vi "Zernike_gen.vi"(8 "Coefficient":dbl[](array[numeric]), 9 "Gray level max":i32=255, 10 "dimension size y":i32=1024, 11 "dimension size x":i32=1280) -> (3 "mask":dbl[][](array[numeric]))   [LabVIEW 2020]
panel:
  out "theta":u8[][](array[numeric])
  out "rho":u8[][](array[numeric])
  out "X":u8[][](array[numeric])
  out "Y":u8[][](array[numeric])
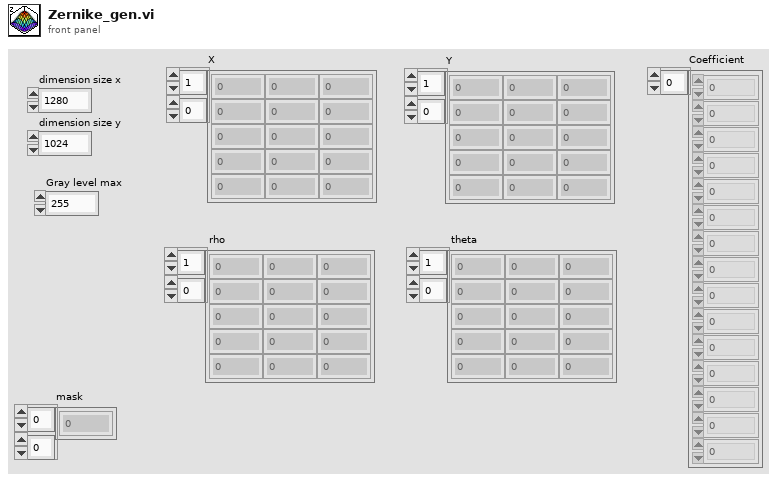
[diagram p1: front panel]
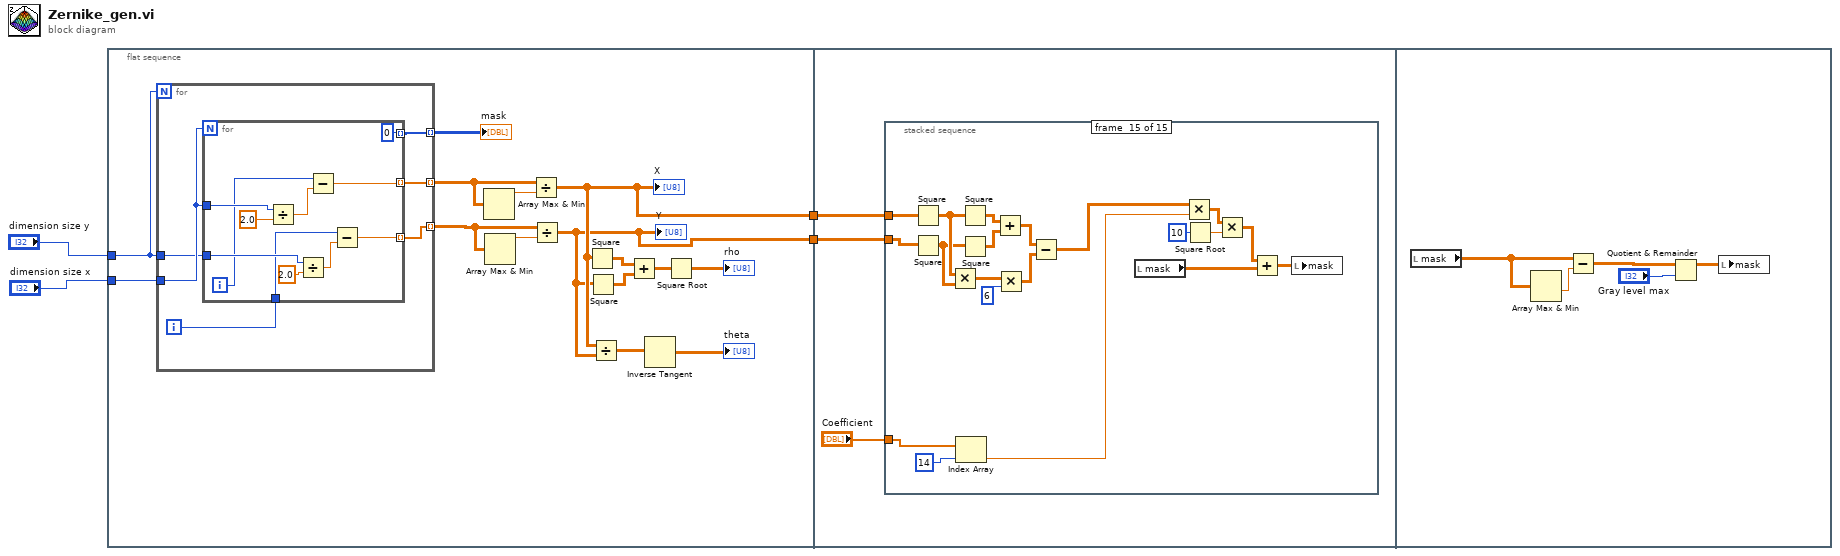
[diagram p0: block diagram]
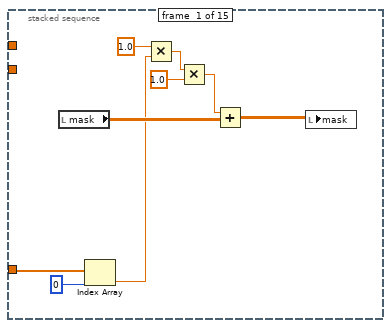
[diagram p2: hidden frame]
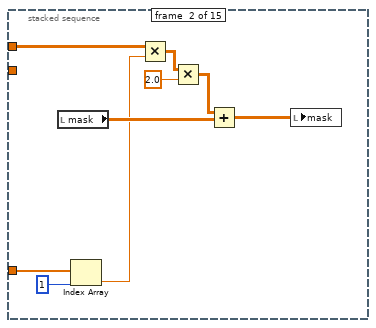
[diagram p3: hidden frame]
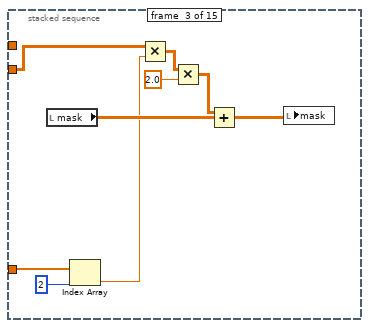
[diagram p4: hidden frame]
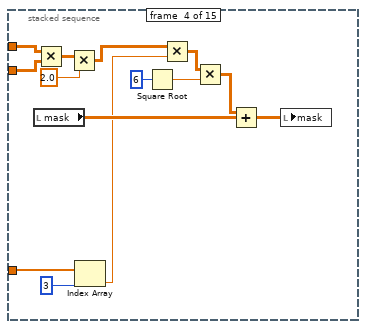
[diagram p5: hidden frame]
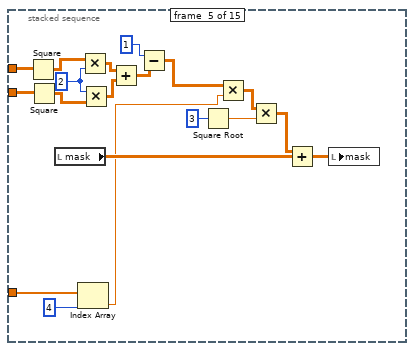
[diagram p6: hidden frame]
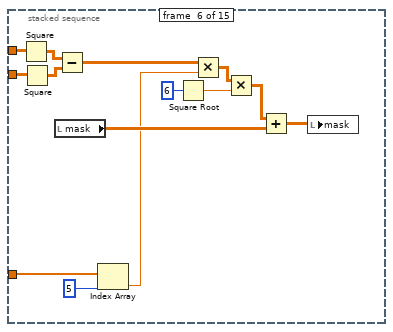
[diagram p7: hidden frame]
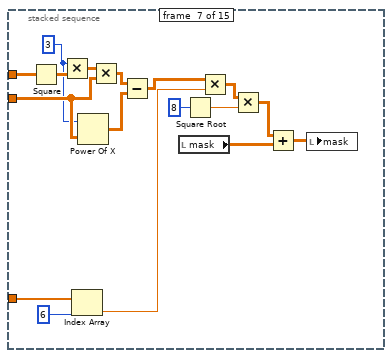
[diagram p8: hidden frame]
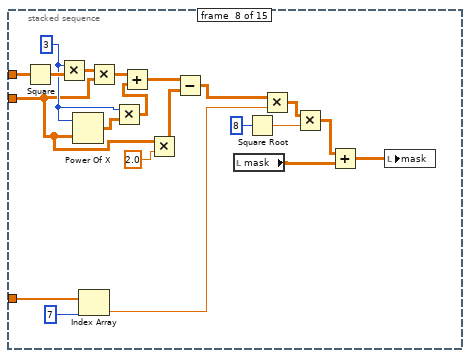
[diagram p9: hidden frame]
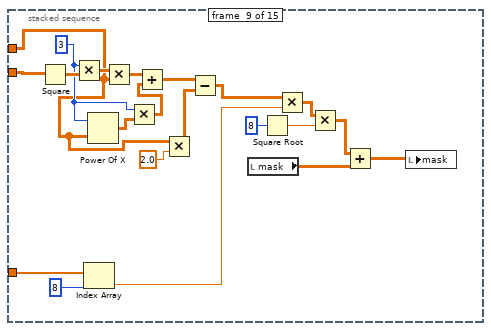
[diagram p10: hidden frame]
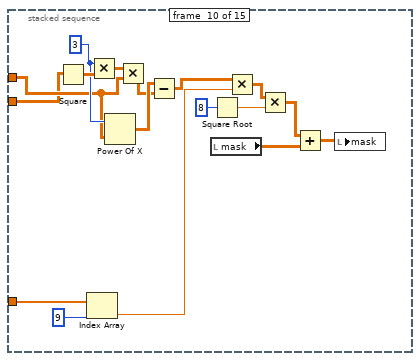
[diagram p11: hidden frame]
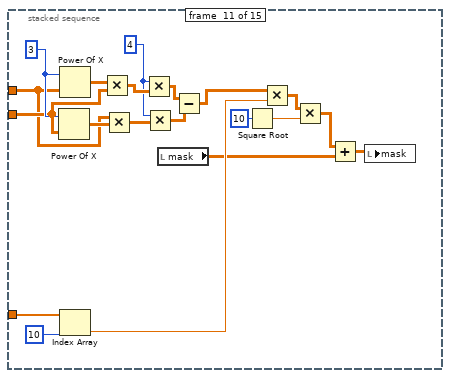
[diagram p12: hidden frame]
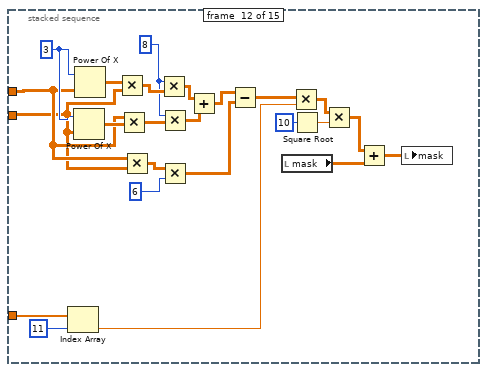
[diagram p13: hidden frame]
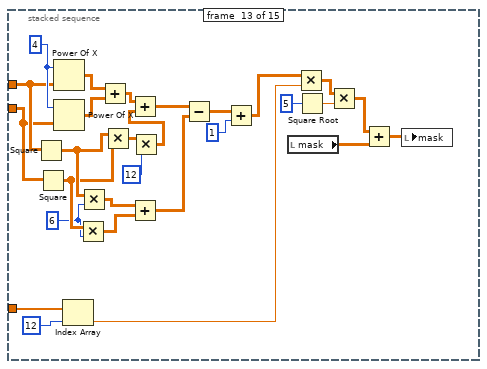
[diagram p14: hidden frame]
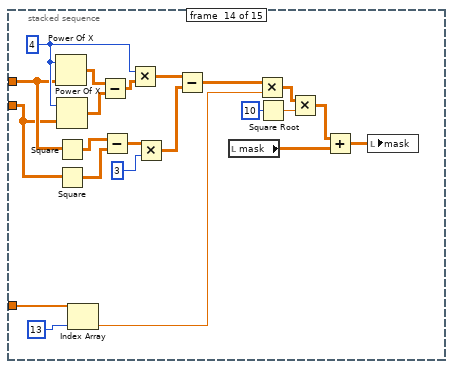
[diagram p15: hidden frame]
diagram:
  n1 = flat-sequence {
    tunnel: [w6] -> w4
    tunnel: [w5] -> w3
    tunnel: "dimension size x" -> [w19]
    tunnel: "dimension size y" -> [w15]
    tunnel: w4 -> [w39]
    tunnel: w3 -> [w37]
    frame #0 {
      n2 = for {
        N: w15 -> [_]
        tunnel: [w25] -> w10 mode=indexing
        tunnel: w19 -> [w22]
        tunnel: [w23] -> w12 mode=indexing
        tunnel: w15 -> [w21]
        tunnel: [w20] -> w9 mode=indexing
        i -> [w24]
        n3 = for {
          N: w22 -> [_]
          tunnel: [w28] -> w25 mode=indexing
          tunnel: w24 -> [w29]
          tunnel: [w33] -> w23 mode=indexing
          tunnel: w22 -> [w35]
          tunnel: w21 -> [w31]
          tunnel: [0] -> w20 mode=indexing
          i -> [w27]
          n4 = Divide(x=w35, y=2.0) -> (x/y=w34:dbl)
          n5 = Divide(x=w31, y=2.0) -> (x/y=w30:dbl)
          n6 = Subtract(x=w27, y=w34) -> (x-y=w33:dbl)
          n7 = Subtract(x=w29, y=w30) -> (x-y=w28:dbl)
        }
      }
      "mask" <- w9
      n8 = Array Max & Min(array=w12) -> (max value=w13:dbl)  [unwired: 3 out]
      n9 = Array Max & Min(array=w10) -> (max value=w11:dbl)  [unwired: 3 out]
      n10 = Divide(x=w12, y=w13) -> (x/y=w6:dbl[][])
      "X" <- w6
      n11 = Divide(x=w10, y=w11) -> (x/y=w5:dbl[][])
      "Y" <- w5
      n12 = Square(x=w6) -> (x^2=w18:dbl[][])
      n13 = Square(x=w5) -> (x^2=w17:dbl[][])
      n14 = Divide(x=w6, y=w5) -> (x/y=w14:dbl[][])
      n15 = Add(x=w18, y=w17) -> (x+y=w16:dbl[][])
      n16 = Inverse Tangent(1:w14) -> (0:→"theta":dbl[][])
      n17 = Square Root(x=w16) -> (sqrt(x)=→"rho":dbl[][])
    }
    frame #1 {
      n18 = stacked-sequence {
        tunnel: w39 -> [_ w53 _ w78 w95 w109 w126 w147 w157 w181 w200 w221 w254 w275 w298]
        tunnel: "Coefficient" -> [w47 w54 w59 w68 w82 w101 w117 w132 w155 w176 w194 w213 w237 w265 w287]
        tunnel: w37 -> [_ _ w61 w77 w94 w108 w122 w139 w158 w180 w203 w220 w253 w274 w297]
        frame #0 {
          n19 = local read "mask"() -> (w43:dbl[][])
          n20 = Index Array(array=w47, index=0) -> (element=w40:dbl)
          n21 = Multiply(x=1.0, y=w40) -> (x*y=w45:dbl)
          n22 = Multiply(x=w45, y=1.0) -> (x*y=w46:dbl)
          n23 = Add(x=w46, y=w43) -> (x+y=w42:dbl[][])
          n24 = local write "mask"(w42) -> ()
        }
        frame #1 {
          n25 = local read "mask"() -> (w55:dbl[][])
          n26 = Index Array(array=w54, index=1) -> (element=w52:dbl)
          n27 = Multiply(x=w53, y=w52) -> (x*y=w50:dbl[][])
          n28 = Multiply(x=w50, y=2.0) -> (x*y=w49:dbl[][])
          n29 = Add(x=w49, y=w55) -> (x+y=w56:dbl[][])
          n30 = local write "mask"(w56) -> ()
        }
        frame #2 {
          n31 = local read "mask"() -> (w63:dbl[][])
          n32 = Index Array(array=w59, index=2) -> (element=w58:dbl)
          n33 = Multiply(x=w61, y=w58) -> (x*y=w65:dbl[][])
          n34 = Multiply(x=w65, y=2.0) -> (x*y=w66:dbl[][])
          n35 = Add(x=w66, y=w63) -> (x+y=w62:dbl[][])
          n36 = local write "mask"(w62) -> ()
        }
        frame #3 {
          n37 = local read "mask"() -> (w71:dbl[][])
          n38 = Multiply(x=w78, y=w77) -> (x*y=w75:dbl[][])
          n39 = Multiply(x=w75, y=2.0) -> (x*y=w74:dbl[][])
          n40 = Index Array(array=w68, index=3) -> (element=w67:dbl)
          n41 = Square Root(x=6) -> (sqrt(x)=w72:dbl)
          n42 = Multiply(x=w74, y=w67) -> (x*y=w80:dbl[][])
          n43 = Multiply(x=w80, y=w72) -> (x*y=w79:dbl[][])
          n44 = Add(x=w79, y=w71) -> (x+y=w70:dbl[][])
          n45 = local write "mask"(w70) -> ()
        }
        frame #4 {
          w91 = 2
          n46 = Square(x=w95) -> (x^2=w93:dbl[][])
          n47 = Square(x=w94) -> (x^2=w92:dbl[][])
          n48 = local read "mask"() -> (w85:dbl[][])
          n49 = Index Array(array=w82, index=4) -> (element=w81:dbl)
          n50 = Multiply(x=w93, y=w91) -> (x*y=w90:dbl[][])
          n51 = Multiply(x=w91, y=w92) -> (x*y=w89:dbl[][])
          n52 = Add(x=w90, y=w89) -> (x+y=w88:dbl[][])
          n53 = Subtract(x=1, y=w88) -> (x-y=w86:dbl[][])
          n54 = Square Root(x=3) -> (sqrt(x)=w99:dbl)
          n55 = Multiply(x=w86, y=w81) -> (x*y=w97:dbl[][])
          n56 = Multiply(x=w97, y=w99) -> (x*y=w98:dbl[][])
          n57 = Add(x=w98, y=w85) -> (x+y=w84:dbl[][])
          n58 = local write "mask"(w84) -> ()
        }
        frame #5 {
          n59 = Square(x=w109) -> (x^2=w107:dbl[][])
          n60 = Square(x=w108) -> (x^2=w106:dbl[][])
          n61 = local read "mask"() -> (w104:dbl[][])
          n62 = Subtract(x=w107, y=w106) -> (x-y=w105:dbl[][])
          n63 = Index Array(array=w101, index=5) -> (element=w100:dbl)
          n64 = Square Root(x=6) -> (sqrt(x)=w111:dbl)
          n65 = Multiply(x=w105, y=w100) -> (x*y=w113:dbl[][])
          n66 = Multiply(x=w113, y=w111) -> (x*y=w112:dbl[][])
          n67 = Add(x=w112, y=w104) -> (x+y=w103:dbl[][])
          n68 = local write "mask"(w103) -> ()
        }
        frame #6 {
          w121 = 3
          n69 = Square(x=w126) -> (x^2=w125:dbl[][])
          n70 = Multiply(x=w121, y=w125) -> (x*y=w124:dbl[][])
          n71 = Index Array(array=w117, index=6) -> (element=w116:dbl)
          n72 = Power Of X(1:w122, 2:w121) -> (0:w120:dbl[][])
          n73 = Multiply(x=w124, y=w122) -> (x*y=w123:dbl[][])
          n74 = Subtract(x=w123, y=w120) -> (x-y=w119:dbl[][])
          n75 = local read "mask"() -> (w115:dbl[][])
          n76 = Square Root(x=8) -> (sqrt(x)=w130:dbl)
          n77 = Multiply(x=w119, y=w116) -> (x*y=w128:dbl[][])
          n78 = Multiply(x=w128, y=w130) -> (x*y=w129:dbl[][])
          n79 = Add(x=w129, y=w115) -> (x+y=w114:dbl[][])
          n80 = local write "mask"(w114) -> ()
        }
        frame #7 {
          w142 = 3
          n81 = Square(x=w147) -> (x^2=w146:dbl[][])
          n82 = Multiply(x=w142, y=w146) -> (x*y=w145:dbl[][])
          n83 = Power Of X(1:w139, 2:w142) -> (0:w143:dbl[][])
          n84 = Index Array(array=w132, index=7) -> (element=w131:dbl)
          n85 = Multiply(x=w145, y=w139) -> (x*y=w144:dbl[][])
          n86 = Multiply(x=w142, y=w143) -> (x*y=w141:dbl[][])
          n87 = Add(x=w144, y=w141) -> (x+y=w137:dbl[][])
          n88 = Multiply(x=w139, y=2.0) -> (x*y=w138:dbl[][])
          n89 = Subtract(x=w137, y=w138) -> (x-y=w136:dbl[][])
          n90 = local read "mask"() -> (w135:dbl[][])
          n91 = Square Root(x=8) -> (sqrt(x)=w151:dbl)
          n92 = Multiply(x=w136, y=w131) -> (x*y=w149:dbl[][])
          n93 = Multiply(x=w149, y=w151) -> (x*y=w150:dbl[][])
          n94 = Add(x=w150, y=w135) -> (x+y=w134:dbl[][])
          n95 = local write "mask"(w134) -> ()
        }
        frame #8 {
          w160 = 3
          n96 = Square(x=w158) -> (x^2=w165:dbl[][])
          n97 = Multiply(x=w160, y=w165) -> (x*y=w166:dbl[][])
          n98 = Index Array(array=w155, index=8) -> (element=w154:dbl)
          n99 = Power Of X(1:w157, 2:w160) -> (0:w168:dbl[][])
          n100 = Multiply(x=w166, y=w157) -> (x*y=w167:dbl[][])
          n101 = Multiply(x=w160, y=w168) -> (x*y=w169:dbl[][])
          n102 = Add(x=w167, y=w169) -> (x+y=w171:dbl[][])
          n103 = Multiply(x=w157, y=2.0) -> (x*y=w170:dbl[][])
          n104 = Subtract(x=w171, y=w170) -> (x-y=w172:dbl[][])
          n105 = local read "mask"() -> (w153:dbl[][])
          n106 = Square Root(x=8) -> (sqrt(x)=w162:dbl)
          n107 = Multiply(x=w172, y=w154) -> (x*y=w164:dbl[][])
          n108 = Multiply(x=w164, y=w162) -> (x*y=w163:dbl[][])
          n109 = Add(x=w163, y=w153) -> (x+y=w152:dbl[][])
          n110 = local write "mask"(w152) -> ()
        }
        frame #9 {
          w182 = 3
          n111 = Square(x=w180) -> (x^2=w187:dbl[][])
          n112 = Index Array(array=w176, index=9) -> (element=w175:dbl)
          n113 = Multiply(x=w182, y=w187) -> (x*y=w188:dbl[][])
          n114 = Power Of X(1:w181, 2:w182) -> (0:w179:dbl[][])
          n115 = Multiply(x=w188, y=w181) -> (x*y=w178:dbl[][])
          n116 = Subtract(x=w179, y=w178) -> (x-y=w189:dbl[][])
          n117 = local read "mask"() -> (w174:dbl[][])
          n118 = Square Root(x=8) -> (sqrt(x)=w184:dbl)
          n119 = Multiply(x=w189, y=w175) -> (x*y=w186:dbl[][])
          n120 = Multiply(x=w186, y=w184) -> (x*y=w185:dbl[][])
          n121 = Add(x=w185, y=w174) -> (x+y=w173:dbl[][])
          n122 = local write "mask"(w173) -> ()
        }
        frame #10 {
          w198 = 4
          w205 = 3
          n123 = Power Of X(1:w203, 2:w205) -> (0:w201:dbl[][])
          n124 = Power Of X(1:w200, 2:w205) -> (0:w204:dbl[][])
          n125 = Index Array(array=w194, index=10) -> (element=w193:dbl)
          n126 = Multiply(x=w204, y=w203) -> (x*y=w202:dbl[][])
          n127 = Multiply(x=w200, y=w201) -> (x*y=w199:dbl[][])
          n128 = Multiply(x=w198, y=w202) -> (x*y=w197:dbl[][])
          n129 = Multiply(x=w198, y=w199) -> (x*y=w192:dbl[][])
          n130 = local read "mask"() -> (w191:dbl[][])
          n131 = Subtract(x=w197, y=w192) -> (x-y=w196:dbl[][])
          n132 = Square Root(x=10) -> (sqrt(x)=w209:dbl)
          n133 = Multiply(x=w196, y=w193) -> (x*y=w207:dbl[][])
          n134 = Multiply(x=w207, y=w209) -> (x*y=w208:dbl[][])
          n135 = Add(x=w208, y=w191) -> (x+y=w190:dbl[][])
          n136 = local write "mask"(w190) -> ()
        }
        frame #11 {
          w222 = 8
          w223 = 3
          n137 = Index Array(array=w213, index=11) -> (element=w212:dbl)
          n138 = Power Of X(1:w220, 2:w223) -> (0:w226:dbl[][])
          n139 = Power Of X(1:w221, 2:w223) -> (0:w224:dbl[][])
          n140 = Multiply(x=w224, y=w220) -> (x*y=w225:dbl[][])
          n141 = Multiply(x=w221, y=w226) -> (x*y=w227:dbl[][])
          n142 = Multiply(x=w221, y=w220) -> (x*y=w218:dbl[][])
          n143 = Multiply(x=w222, y=w225) -> (x*y=w228:dbl[][])
          n144 = Multiply(x=w222, y=w227) -> (x*y=w229:dbl[][])
          n145 = Multiply(x=w218, y=6) -> (x*y=w216:dbl[][])
          n146 = Add(x=w228, y=w229) -> (x+y=w217:dbl[][])
          n147 = Subtract(x=w217, y=w216) -> (x-y=w215:dbl[][])
          n148 = local read "mask"() -> (w211:dbl[][])
          n149 = Multiply(x=w215, y=w212) -> (x*y=w233:dbl[][])
          n150 = Square Root(x=10) -> (sqrt(x)=w231:dbl)
          n151 = Multiply(x=w233, y=w231) -> (x*y=w232:dbl[][])
          n152 = Add(x=w232, y=w211) -> (x+y=w210:dbl[][])
          n153 = local write "mask"(w210) -> ()
        }
        frame #12 {
          w246 = 6
          w257 = 4
          n154 = Square(x=w254) -> (x^2=w248:dbl[][])
          n155 = Square(x=w253) -> (x^2=w247:dbl[][])
          n156 = Power Of X(1:w254, 2:w257) -> (0:w256:dbl[][])
          n157 = Power Of X(1:w253, 2:w257) -> (0:w255:dbl[][])
          n158 = Index Array(array=w237, index=12) -> (element=w236:dbl)
          n159 = Multiply(x=w247, y=w246) -> (x*y=w244:dbl[][])
          n160 = Multiply(x=w248, y=w246) -> (x*y=w245:dbl[][])
          n161 = Add(x=w256, y=w255) -> (x+y=w252:dbl[][])
          n162 = Multiply(x=w248, y=w247) -> (x*y=w251:dbl[][])
          n163 = Add(x=w245, y=w244) -> (x+y=w242:dbl[][])
          n164 = Multiply(x=w251, y=12) -> (x*y=w249:dbl[][])
          n165 = Add(x=w252, y=w249) -> (x+y=w243:dbl[][])
          n166 = Subtract(x=w243, y=w242) -> (x-y=w240:dbl[][])
          n167 = Add(x=w240, y=1) -> (x+y=w239:dbl[][])
          n168 = local read "mask"() -> (w235:dbl[][])
          n169 = Multiply(x=w239, y=w236) -> (x*y=w259:dbl[][])
          n170 = Square Root(x=5) -> (sqrt(x)=w261:dbl)
          n171 = Multiply(x=w259, y=w261) -> (x*y=w260:dbl[][])
          n172 = Add(x=w260, y=w235) -> (x+y=w234:dbl[][])
          n173 = local write "mask"(w234) -> ()
        }
        frame #13 {
          w276 = 4
          n174 = Power Of X(1:w275, 2:w276) -> (0:w279:dbl[][])
          n175 = Power Of X(1:w274, 2:w276) -> (0:w278:dbl[][])
          n176 = Square(x=w275) -> (x^2=w273:dbl[][])
          n177 = Square(x=w274) -> (x^2=w272:dbl[][])
          n178 = Index Array(array=w265, index=13) -> (element=w264:dbl)
          n179 = Subtract(x=w279, y=w278) -> (x-y=w277:dbl[][])
          n180 = Subtract(x=w273, y=w272) -> (x-y=w271:dbl[][])
          n181 = Multiply(x=w276, y=w277) -> (x*y=w269:dbl[][])
          n182 = Multiply(x=w271, y=3) -> (x*y=w268:dbl[][])
          n183 = Subtract(x=w269, y=w268) -> (x-y=w267:dbl[][])
          n184 = local read "mask"() -> (w263:dbl[][])
          n185 = Multiply(x=w267, y=w264) -> (x*y=w283:dbl[][])
          n186 = Square Root(x=10) -> (sqrt(x)=w281:dbl)
          n187 = Multiply(x=w283, y=w281) -> (x*y=w282:dbl[][])
          n188 = Add(x=w282, y=w263) -> (x+y=w262:dbl[][])
          n189 = local write "mask"(w262) -> ()
        }
        frame #14 {
          n190 = Square(x=w298) -> (x^2=w296:dbl[][])
          n191 = Square(x=w297) -> (x^2=w295:dbl[][])
          n192 = Multiply(x=w296, y=w295) -> (x*y=w294:dbl[][])
          n193 = Index Array(array=w287, index=14) -> (element=w286:dbl)
          n194 = Square(x=w296) -> (x^2=w293:dbl[][])
          n195 = Square(x=w295) -> (x^2=w292:dbl[][])
          n196 = Add(x=w293, y=w292) -> (x+y=w291:dbl[][])
          n197 = Multiply(x=w294, y=6) -> (x*y=w290:dbl[][])
          n198 = Subtract(x=w291, y=w290) -> (x-y=w289:dbl[][])
          n199 = local read "mask"() -> (w285:dbl[][])
          n200 = Multiply(x=w289, y=w286) -> (x*y=w303:dbl[][])
          n201 = Square Root(x=10) -> (sqrt(x)=w301:dbl)
          n202 = Multiply(x=w303, y=w301) -> (x*y=w302:dbl[][])
          n203 = Add(x=w302, y=w285) -> (x+y=w284:dbl[][])
          n204 = local write "mask"(w284) -> ()
        }
      }
    }
    frame #2 {
      n205 = local read "mask"() -> (w307:dbl[][])
      n206 = Array Max & Min(array=w307) -> (min value=w306:dbl)  [unwired: 3 out]
      n207 = Subtract(x=w307, y=w306) -> (x-y=w305:dbl[][])
      n208 = Quotient & Remainder(x=w305, y="Gray level max") -> (x-y*floor(x/y)=w304:dbl[][])  [unwired: 1 out]
      n209 = local write "mask"(w304) -> ()
    }
  }
